vi "publishGrating.vi"(8 "error in (no error)":errorcluster, 10 "GratingType":T1=enum."Red", 11 "Monochromator in":refnum<class "Monochromator.lvclass">) -> (0 "error out":errorcluster, 3 "Monochromator out":refnum<class "Monochromator.lvclass">)   [LabVIEW 2016, in "Monochromator.lvclass"]
uses:
  Monochromator.lvclass
  Typedefs/GratingType.ctl
  Monochromator.lvclass/Monochromator.ctl
  MonoPubSubData/MonoPubSubData.lvclass/MonoPubSubData.ctl
  MonoPubSubData/MonoPubSubData.lvclass
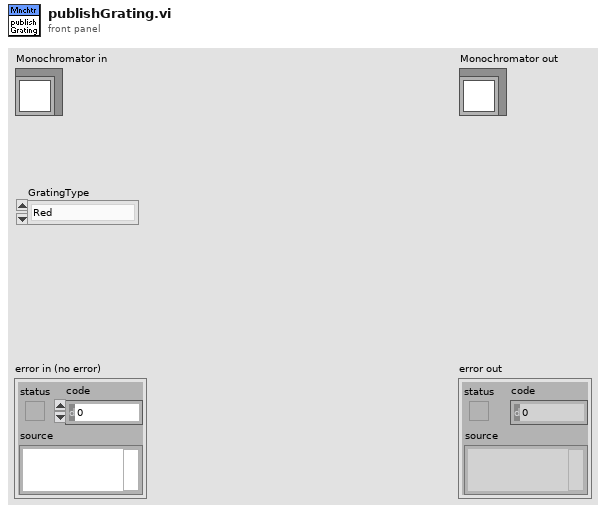
[diagram p1: front panel]
types:
  T1 = typedef "GratingType.ctl" = enum16{"Blue", "Red", "Mirror"}
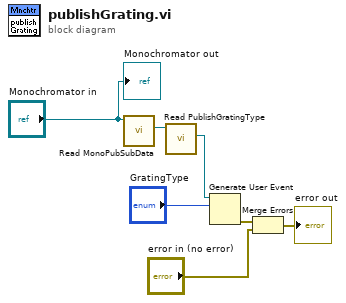
[diagram p0: block diagram]
diagram:
  n1 = call "Read MonoPubSubData.vi"("Monochromator in"="Monochromator in") -> ("MonoPubSubData.lvclass"=w5:refnum<class "MonoPubSubData.lvclass">)  [unwired: 8 in, 2 out]
  n2 = call "Read PublishGratingType.vi"("MonoPubSubData in"=w5) -> ("PublishGratingType"=w4:refnum<user-event>)  [unwired: 8 in, 2 out]
  n3 = Generate User Event(user event=w4, event data cluster="GratingType") -> (error out=w3:errorcluster)  [unwired: 2 in, 1 out]
  n4 = Merge Errors(w3, "error in (no error)") -> (→"error out":errorcluster)
  "Monochromator out" <- "Monochromator in"
